vi "mmap.vi"(6 "process (shared)":T1, 7 "protections (read/write)":T2={"read"=TRUE, "write"=TRUE, "execute"=FALSE}, 8 "error in (no error)":errorcluster, 9 "offset (0)":u64, 10 "number of bytes":u64, 11 "file descriptor":i32) -> (0 "error out":errorcluster, 2 "pointer":u64 format="0x%016x", 3 "file descriptor":i32)   [LabVIEW 2013, in "Shared Memory.lvlib" / "Shared Memory.lvclass"]
doc: "Wrapper VI for Linux function mmap()."
uses:
  Shared Memory.lvclass
  Public/Controls/permissions.ctl
  Public/Controls/mman sharing.ctl
  Controls/functions.ctl
  <vilib>/NI/NI Linux RT Errno/Linux Errno.lvlib
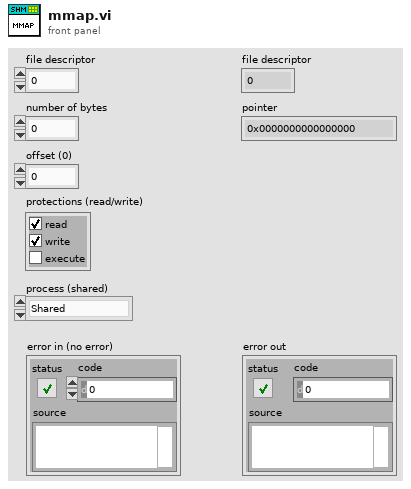
[diagram p1: front panel]
types:
  T1 = typedef "Shared Memory.lvlib/Shared Memory.lvclass/mman sharing.ctl" = enum16{"Shared", "Private"}
  T2 = typedef "Shared Memory.lvlib/Shared Memory.lvclass/permissions.ctl" = cluster{"read":bool, "write":bool, "execute":bool}
  T3 = typedef "Shared Memory.lvlib/Shared Memory.lvclass/functions.ctl" = enum16{"unspecified", "shm_open", "ftruncate", "mmap", "munmap", "close", "shm_unlink", "fstat"}
  T4 = typedef "Linux Errno.lvlib/errno.ctl" = enum16{"NO ERROR", "EPERM", "ENOENT", "ESRCH", "EINTR", "EIO", "ENXIO", "E2BIG", "ENOEXEC", "EBADF", "ECHILD", "EAGAIN", "ENOMEM", "EACCES", "EFAULT", "ENOTBLK", "EBUSY", "EEXIST", "EXDEV", "ENODEV", "ENOTDIR", "EISDIR", "EINVAL", "ENFILE", "EMFILE", "ENOTTY", "ETXTBSY", "EFBIG", "ENOSPC", "ESPIPE", "EROFS", "EMLINK", "EPIPE", "EDOM", "ERANGE", "EDADLK", "ENAMETOOLONG", "ENOLCK", "ENOSYS", "ENOTEMPTY", "ELOOP", "EWOULDBLOCK", "ENOMSG", "EIDRM", "ECHRNG", "EL2NSYNC", "EL3HLT", "EL3RST", "ELNRNG", "EUNATCH", "ENOCSI", "EL2HLT", "EBADE", "EBADR", "EXFULL", "ENOANO", "EBADRQC", "EBADSLT", "EDEADLOCK", "EBFONT", "ENOSTR", "ENODATA", "ETIME", "ENOSR", "ENONET", "ENOPKG", "EREMOTE", "ENOLINK", "EADV", "ESRMNT", "ECOMM", "EPROTO", "EMULTIHOP", "EDOTDOT", "EBADMSG", "EOVERFLOW", "ENOTUNIQ", "EBADFD", "EREMCHG", "ELIBACC", "ELIBBAD", "ELIBSCN", "ELIBMAX", "ELIBEXEC", "ELISEQ", "ERESTART", "ESTRPIPE", "EUSERS", "ENOTSOCK", "EDESTADDRREQ", "EMSGSIZE", "EPROTOTYPE", "ENOPROTOOPT", "EPROTONOSUPPORT", "ESOCKTNOSUPPORT", "EOPNOTSUPP", "EPFNOSUPPORT", "EAFNOSUPPORT", "EADDRINUSE", "EADDRNOTAVAIL", "ENETDOWN", "ENETUNREACH", "ENETRESET", "ECONNABORTED", "ECONNRESET", "ENOBUFS", "EISCONN", "ENOTCONN", "ESHUTDOWN", "ETOOMANYREFS", "ETIMEDOUT", "ECONNREFUSED", "EHOSTDOWN", "EHOSTUNREACH", "EALREADY", "EINPROGRESS", "ESTALE", "EUCLEAN", "ENOTNAM", "ENAVAIL", "EISNAM", "EREMOTEIO", "EDQUOT", "ENOMEDIUM", "EMEDIUMTYPE", "ECANCELED", "ENOKEY", "EKEYEXPIRED", "EKEYREVOKED", "EKEYREJECTED", "EOWNERDEAD", "ENOTRECOVERABLE", "ERFKILL", "EHWPOISON", "UNDEFINED"}
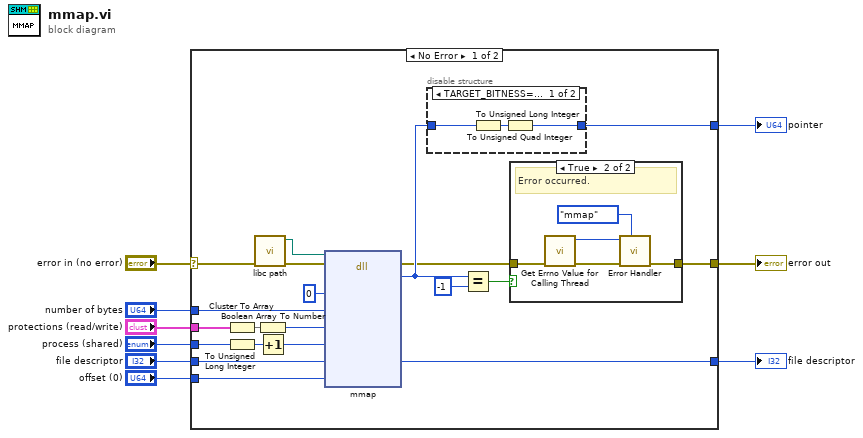
[diagram p0: block diagram]
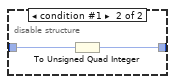
[diagram p3: hidden frame]
diagram:
  n1 = case shown="No Error" "error in (no error)" {
    selector: "error in (no error)" -> [w24 w42]
    tunnel: "file descriptor" -> [w29 w41]
    tunnel: [w11 w42] -> w8
    tunnel: [w28 w41] -> w7
    tunnel: "offset (0)" -> [w27 _]
    tunnel: [w26 _] -> w4
    tunnel: "number of bytes" -> [w25 _]
    tunnel: "protections (read/write)" -> [w23 _]
    tunnel: "process (shared)" -> [w22 _]
    frame No Error {
      n2 = Cluster To Array(cluster=w23) -> (array=w19:bool[])
      n3 = To Unsigned Long Integer(number=w22) -> (unsigned 32bit integer=w18:u32)
      n4 = call "libc path.vi"("error in (no error)"=w24) -> ("error out"=w20:errorcluster, "path to libc"=w21:path)  [unwired: 9 in]
      n5 = Boolean Array To Number(Boolean array=w19) -> (number=w16:u32)
      n6 = Increment(x=w18) -> (x+1=w15:u32)
      n7 = dll-call lib="?" fn="mmap"(path in=w21, error in=w20, "addr"=u64 0, "size"=w25, "prot"=w16, "flags"=w15, "fd"=w29, "offset"=w27) -> (error out=w12:errorcluster, "pointer"=w13:i64, "fd"=w28:i32)  [unwired: 6 in, 1 out]
      n8 = disable-structure shown="TARGET_BITNESS==32" {
        disable-tunnel: w13 -> [w36 w40]
        disable-tunnel: [w38 w39] -> w26
        frame condition #0 (active) {
          n9 = To Unsigned Long Integer(number=w36) -> (unsigned 32bit integer=w37:u32)
          n10 = To Unsigned Quad Integer(1:w37) -> (0:w38:u64)
        }
        frame condition #1 {
          n11 = To Unsigned Quad Integer(1:w40) -> (0:w39:u64)
        }
      }
      n12 = Equal?(x=w13, y=i64 -1) -> (x = y?=w10:bool)
      n13 = case shown="True" w10 {
        tunnel: w12 -> [w30 w35]
        tunnel: [w30 w32] -> w11
        frame False {
          # "No error."
        }
        frame True {
          # "Error occurred."
          n14 = call <vilib>:"Get Errno Value for Calling Thread.vi"("error in (no error)"=w35) -> ("error out"=w33:errorcluster, "errno"=w31:T4)  [unwired: 9 in]
          n15 = call "Error Handler.vi"("function"=functions."mmap", "error in (no error)"=w33, "errno"=w31) -> ("error out"=w32:errorcluster)  [unwired: 8 in]
        }
      }
    }
    frame Error {
    }
  }
  "error out" <- w8
  "file descriptor" <- w7
  "pointer" <- w4
